vi "Serve Web Root.vi"() -> ()   [LabVIEW 2020]
uses:
  <vilib>/IlluminatedG/IG HTTP Server/HTTP Server/Trace Log.ctl
  <vilib>/IlluminatedG/IG HTTP Server/HTTP Server/Trace Item.ctl
  <vilib>/IlluminatedG/IG HTTP Server/HTTP Server/Processing Step.ctl
  <vilib>/IlluminatedG/IG HTTP Utils/HTTP Utils/Method.ctl
  <vilib>/IlluminatedG/IG HTTP Server/HTTP Server/Server Caching.ctl
  <vilib>/IlluminatedG/IG HTTP Server/HTTP Server/StandardFileServe/StandardFileServe.lvclass
  C:/Program Files (x86)/National Instruments/LabVIEW 2020/vi.lib/IlluminatedG/IG HTTP Server/HTTP Server/Handler/Handler.lvclass
  <vilib>/IlluminatedG/IG HTTP Server/HTTP Server/Server/Add Connection Handler.vi
  <vilib>/IlluminatedG/IG HTTP Server/HTTP Server/Server/Add Request Handler.vi
  <vilib>/IlluminatedG/IG HTTP Server/HTTP Server/Server/Add Route Handler.vi
  <vilib>/IlluminatedG/IG HTTP Server/HTTP Server/Server/Add Controller Handler.vi
  <vilib>/IlluminatedG/IG HTTP Server/HTTP Server/Server/Add Controller.vi
  <vilib>/IlluminatedG/IG HTTP Server/HTTP Server/Server/Add Response Handler.vi
  <vilib>/IlluminatedG/IG HTTP Server/HTTP Server/Server/Add Complete Handler.vi
  <vilib>/IlluminatedG/IG HTTP Server/HTTP Server/Server/Add Exception Handler.vi
  <vilib>/IlluminatedG/IG HTTP Server/HTTP Server/Connection Handler/Connection Handler.lvclass
  <vilib>/IlluminatedG/IG HTTP Server/HTTP Server/Request Handler/Request Handler.lvclass
  <vilib>/IlluminatedG/IG HTTP Server/HTTP Server/Route Handler/Route Handler.lvclass
  <vilib>/IlluminatedG/IG HTTP Server/HTTP Server/Controller Handler/Controller Handler.lvclass
  <vilib>/IlluminatedG/IG HTTP Server/HTTP Server/Controller/Controller.lvclass
  <vilib>/IlluminatedG/IG HTTP Server/HTTP Server/Response Handler/Response Handler.lvclass
  <vilib>/IlluminatedG/IG HTTP Server/HTTP Server/Complete Handler/Complete Handler.lvclass
  <vilib>/IlluminatedG/IG HTTP Server/HTTP Server/Exception Handler/Exception Handler.lvclass
  <vilib>/IlluminatedG/IG HTTP Server/HTTP Server/Server/Server.lvclass
  <vilib>/IlluminatedG/IG HTTP Server/HTTP Server/Handler/Handler.lvclass
  <vilib>/IlluminatedG/IG HTTP Server/HTTP Server/RequestTraceLog/RequestTraceLog.lvclass
  <vilib>/IlluminatedG/IG HTTP Server/HTTP Server/HTTP Server.lvlib
  <vilib>/IlluminatedG/IG HTTP Utils/HTTP Utils/HTTP Utils.lvlib
panel:
  in  "Debug":bool=TRUE
  in  "Refresh Traces":bool
  out "Traces":T1[](array[typedef]) {"Sending" format="%_6f"; "Expires" format="%<%X %x>T"; "Created" format="%<%X %x>T"; "Waiting" format="%_6f"; "Parsing" format="%_6f"; "Processing" format="%_6f"; "Items"."Time" format="%.6f"; "Items"."Duration" format="%.6f"}
  out "error out":errorcluster
  in  "Port":u16=36987
  # "Request"
  # "Response"
  # "Session"
  # "Auth"
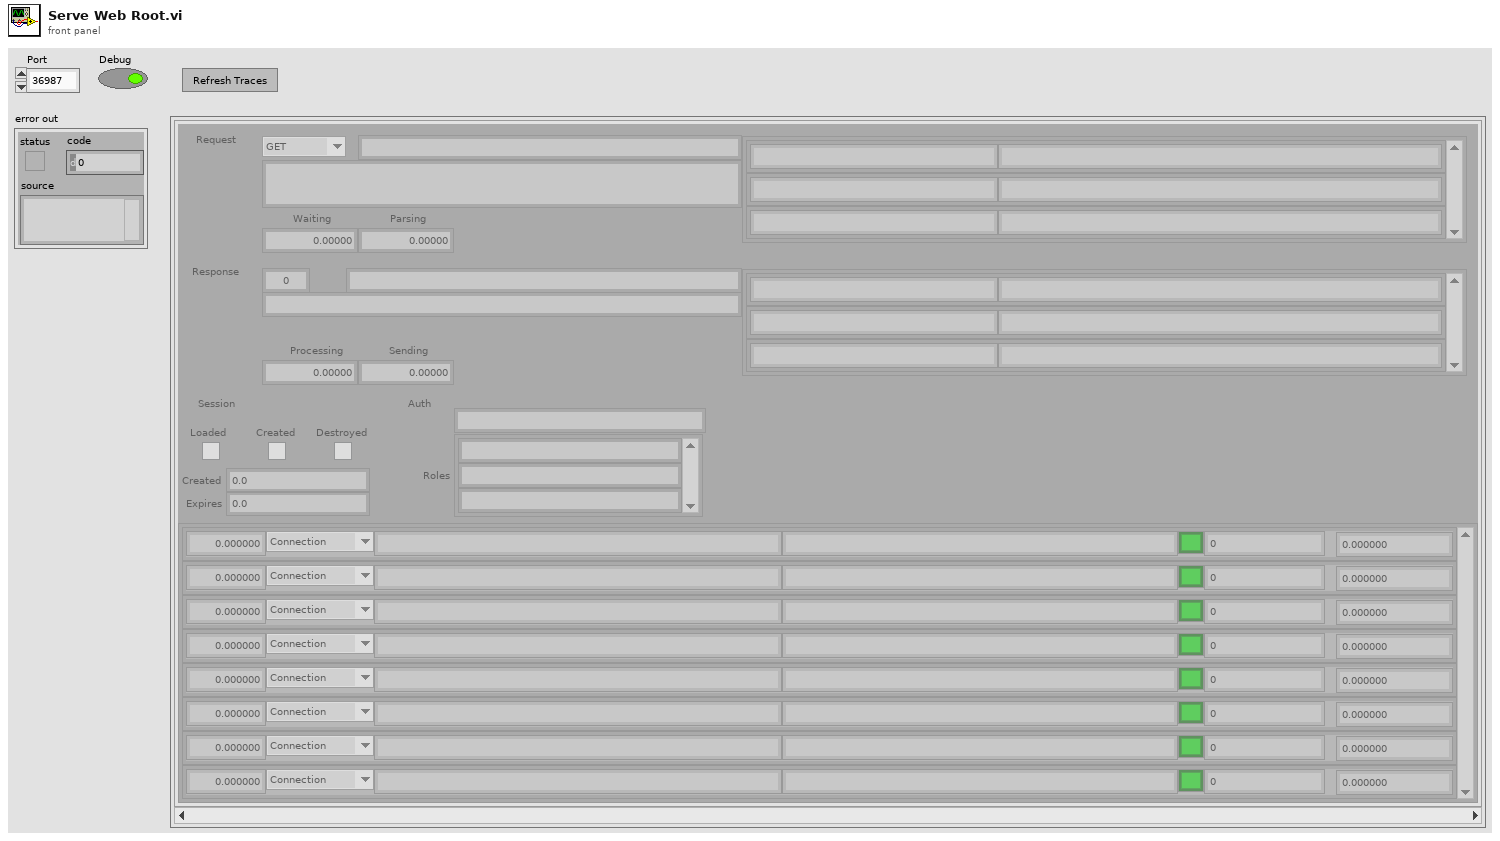
[diagram p1: front panel]
types:
  T1 = typedef "HTTP Server.lvlib/Trace Log.ctl" = cluster{"Items":T2[], "Client":string, "Target":string, "Response Type":string, "Processing":dbl, "Status":u16, "Method":T4, "Content Type":string, "Request Headers":cluster{"Name":string, "Value":string}[], "Parsing":dbl, "Waiting":dbl, "Identity":string, "Loaded":bool, "Created":bool, "Destroyed":bool, "Response Headers":cluster{"Name":string, "Value":string}[], "Created":dbl, "Expires":dbl, "Roles":string[], "Sending":dbl}
  T2 = typedef "HTTP Server.lvlib/Trace Item.ctl" = cluster{"Duration":dbl, "Step":T3, "Class":string, "Info":string, "Status":bool, "Code":i32, "Time":dbl}
  T3 = typedef "HTTP Server.lvlib/Processing Step.ctl" = enum16{"Connection", "Request", "Routing", "Controller Init", "Controller", "Response", "Complete", "Exception"}
  T4 = typedef "HTTP Utils.lvlib/Method.ctl" = enum16{"GET", "HEAD", "POST", "PUT", "DELETE", "CONNECT", "OPTIONS", "TRACE", "PATCH"}
  T5 = typedef "HTTP Server.lvlib/Server Caching.ctl" = cluster{"Auto Cache Static Files":bool, "Cache Folder":path, "Memory Caching Bytes Limit":i32, "Memory Caching Age Limit":dbl, "File Caching Age Limit":dbl, "Default Cache Max Age":i32}
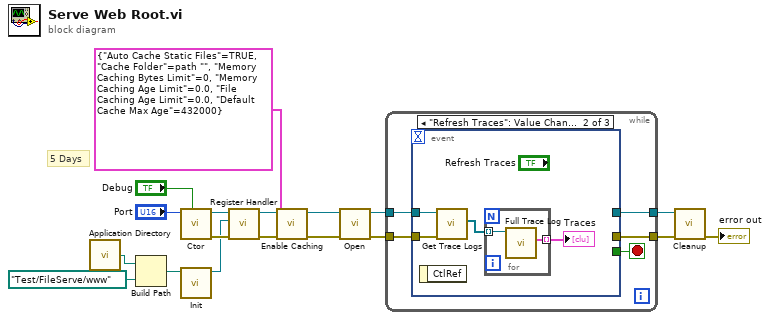
[diagram p0: block diagram]
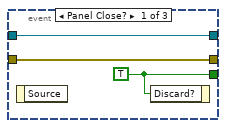
[diagram p2: hidden frame]
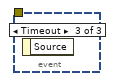
[diagram p3: hidden frame]
diagram:
  # "5 Days"
  n1 = call <vilib>:"Application Directory.vi"() -> ("Application Directory"=w12:path)
  n2 = Build Path(base path=w12, name or relative path=path "Test/FileServe/www") -> (appended path=w10:path)
  n3 = call <vilib>:"Ctor.vi"("Debug (F)"="Debug", "HTTP Port (80)"="Port") -> ("error out"=w7:errorcluster, "Server out"=w8:refnum<class "Server.lvclass">)  [unwired: 8 in]
  n4 = call <vilib>:"Init.vi"("Public Root"=w10) -> ("StandardFileServe out"=w6:refnum<class "StandardFileServe.lvclass">)  [unwired: 9 in, 1 out]
  n5 = call <vilib>:"Register Handler.vi"("error in (no error)"=w7, "Handler"=w6, "Server in"=w8) -> ("error out"=w4:errorcluster, "Server out"=w5:refnum<class "Server.lvclass">)  [unwired: 7 in]
  n6 = call <vilib>:"Enable Caching.vi"("error in (no error)"=w4, "Server Caching"=T5 {"Auto Cache Static Files"=TRUE, "Cache Folder"=path "", "Memory Caching Bytes Limit"=0, "Memory Caching Age Limit"=0.0, "File Caching Age Limit"=0.0, "Default Cache Max Age"=432000}, "Server in"=w5) -> ("error out"=w2:errorcluster, "Server out"=w3:refnum<class "Server.lvclass">)  [unwired: 7 in]
  n7 = call <vilib>:"Open.vi"("error in (no error)"=w2, "Server in"=w3) -> ("error out"=w16:errorcluster, "Server out"=w17:refnum<class "Server.lvclass">)  [unwired: 8 in]
  n8 = while {
    tunnel: w17 -> [w21]
    tunnel: w16 -> [w22]
    tunnel: [w20] -> w15
    tunnel: [w19] -> w14
    stop <- w23 stop-if-true
    n9 = event shown="[1] \"Refresh Traces\": Value Change" {
      selector: _ -> [_ _ _]
      dyn-events: _ -> [_ _ _]
      timeout: _ -> [_ _ _]
      tunnel: [w24 _ _] -> w23
      tunnel: w22 -> [w25 w29 _]
      tunnel: w21 -> [w26 w30 _]
      tunnel: [w26 _ _] -> w20
      tunnel: [w25 _ _] -> w19
      event Panel Close? {
        w24 = TRUE ("Discard?")
        n10 = event-data() -> ()  [unwired: 1 in, 1 out]
        n11 = event-data("Discard?"=w24) -> ()  [unwired: 1 in, 1 out]
      }
      event "Refresh Traces": Value Change {
        n12 = event-data() -> ()  [unwired: 1 in, 1 out]
        n13 = call <vilib>:"Get Trace Logs.vi"("error in (no error)"=w29, "Server in"=w30) -> ("Trace Logs"=w28:refnum<class "RequestTraceLog.lvclass">[])  [unwired: 7 in, 2 out]
        n14 = for {
          tunnel: w28 -> [w32] mode=indexing
          tunnel: [w31] -> w27 mode=indexing
          n15 = call <vilib>:"Full Trace Log.vi"("RequestTraceLog in"=w32) -> ("Trace Log"=w31:T1)  [unwired: 8 in, 2 out]
        }
        "Traces" <- w27
      }
      event Timeout {
        n16 = event-data() -> ()  [unwired: 1 in, 1 out]
      }
    }
  }
  n17 = call <vilib>:"Cleanup.vi"("error in (no error)"=w14, "Server in"=w15) -> ("error out"=→"error out":errorcluster)  [unwired: 9 in]
